vi "ft_data.vi"() -> ()   [LabVIEW 2012]
uses:
  <vilib>/Utility/miscctls.llb/LVDateTimeRec.ctl
  <vilib>/addons/database/Connection.llb/DB Tools Open Connec (String).vi
  <vilib>/addons/database/NI_Database_API.lvlib
panel:
  in  "Data":T1={"query type"="automatic", "device name"="mydevice", "Numeric"=0.0}
  in  "table":string
  out "error out":errorcluster
  out "Array 8":timestamp[](array[timestamp])
  in  "date time rec":T2
  out "Array":string[](array[string])
  in  "path":path=path "c:/"
  out "filenames":string[](array[string])
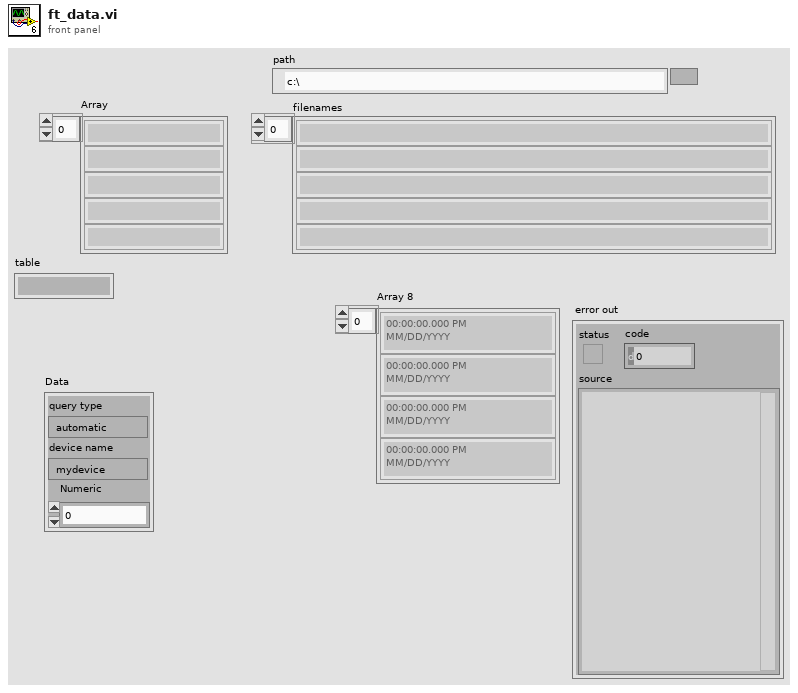
[diagram p1: front panel]
types:
  T1 = cluster{"query type":string, "device name":string, "Numeric":dbl}
  T2 = typedef "LVDateTimeRec.ctl" = cluster{"fractional second":dbl, "second":i32, "minute":i32, "hour":i32, "day of month":i32, "month":i32, "year":i32, "day of week":i32, "day of year":i32, "DST":i32}
  T3 = typedef "NI_Database_API.lvlib/Conn ObjectReference.ctl" = refnum<k1>
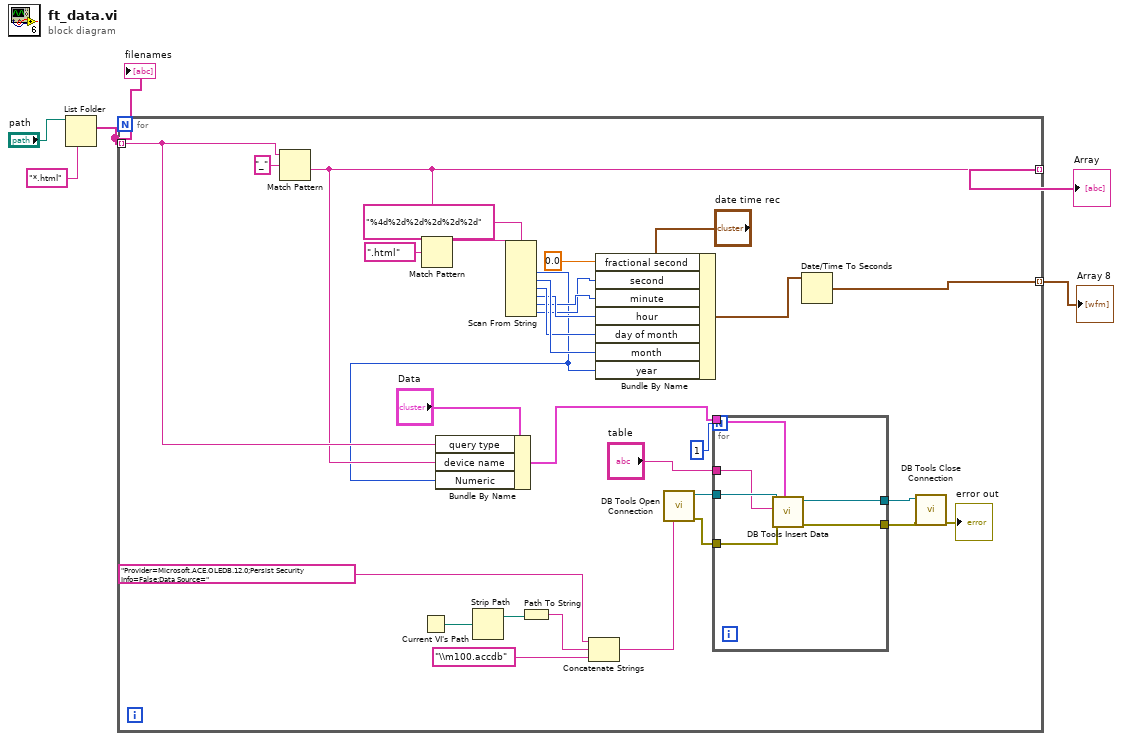
[diagram p0: block diagram]
diagram:
  n1 = List Folder(path="path", pattern="*.html") -> (filenames=w3:string[])  [unwired: 2 in, 3 out]
  "filenames" <- w3
  n2 = for {
    tunnel: w3 -> [w8] mode=indexing
    tunnel: [w7] -> w2 mode=indexing
    tunnel: [w24] -> w1 mode=indexing
    n3 = Match Pattern(string=w8, regular expression="_") -> (after substring=w7:string)  [unwired: 1 in, 3 out]
    n4 = Current VI's Path() -> (path=w22:path)
    n5 = Match Pattern(string=w7, regular expression=".html") -> (before substring=w34:string)  [unwired: 1 in, 3 out]
    n6 = Strip Path(path=w22) -> (stripped path=w20:path)  [unwired: 1 out]
    n7 = Scan From String(format string="%4d%2d%2d%2d%2d%2d", input string=w34) -> (output 1=w6:i32, output 2=w30:i32, output 3=w29:i32, output 4=w28:i32, output 5=w27:i32, output 6=w26:i32)  [unwired: 8 in, 3 out]
    n8 = Bundle By Name(cluster="Data", "query type"=w8, "device name"=w7, "Numeric"=w6) -> (w9:T1)
    n9 = Path To String(path=w20) -> (string=w19:string)
    n10 = Concatenate Strings("Provider=Microsoft.ACE.OLEDB.12.0;Persist Security Info=False;Data Source=", w19, "\\m100.accdb") -> (w17:string)
    n11 = Bundle By Name(cluster="date time rec", "fractional second"=0.0, "second"=w26, "minute"=w27, "hour"=w28, "day of month"=w29, "month"=w30, "year"=w6) -> (w25:T2)
    n12 = call-poly <vilib>:"DB Tools Open Connection.vi"("connection information"=w17) -> ("error out"=w13:errorcluster, "connection reference"=w16:T3)  [unwired: 7 in]
    n13 = for {
      N: 1 -> [_]
      tunnel: w16 -> [w42]
      tunnel: [w41] -> w15
      tunnel: [w40] -> w14
      tunnel: w13 -> [w39]
      tunnel: "table" -> [w38]
      tunnel: w9 -> [w37]
      n14 = call <vilib>:"DB Tools Insert Data.vi"("data"=w37, "error in (no error)"=w39, "table"=w38, "connection reference"=w42) -> ("error out"=w40:errorcluster, "connection reference out"=w41:T3)  [unwired: 6 in]
    }
    n15 = Date/Time To Seconds(2:w25) -> (0:w24:timestamp)  [unwired: 1 in]
    n16 = call <vilib>:"DB Tools Close Connection.vi"("error in (no error)"=w14, "connection reference"=w15) -> ("error out"=→"error out":errorcluster)  [unwired: 5 in]
  }
  "Array" <- w2
  "Array 8" <- w1
